vi "Data Manager.vi"(0 "Max Av Values In":dbl[](array[numeric]), 1 "Data Array In":dbl[][](array[numeric]), 3 "Data":dbl[](array[numeric]), 4 "Is PAT Test?":bool) -> (6 "Max Av Values Out":dbl[](array[numeric]), 7 "Data Array Out":dbl[][](array[numeric]))   [LabVIEW 2018]
uses:
  <vilib>/Analysis/baseanly.llb/Mean (DBL).vi
  <vilib>/Analysis/NI_AALBase.lvlib
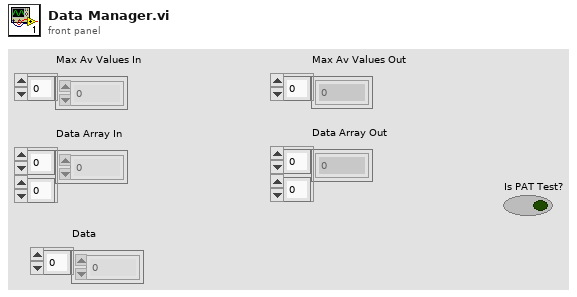
[diagram p1: front panel]
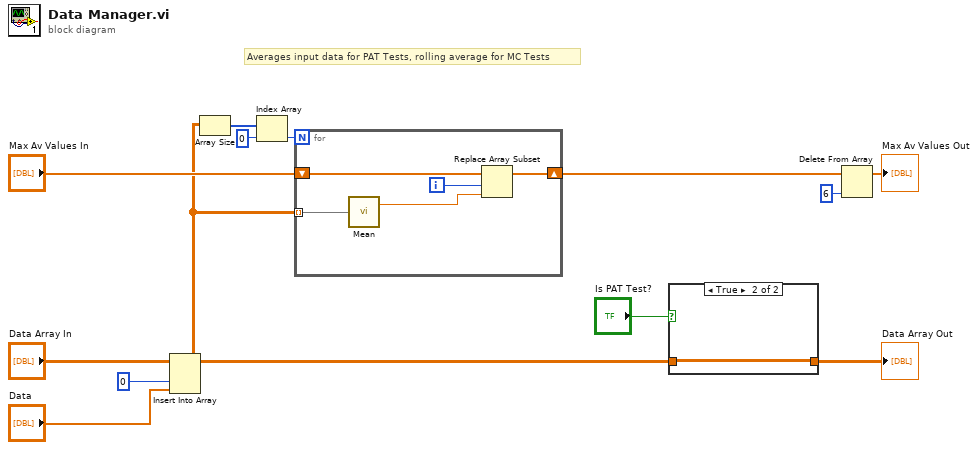
[diagram p0: block diagram]
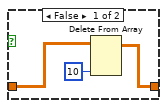
[diagram p2: hidden frame]
diagram:
  # "Averages input data for PAT Tests, rolling average for MC Tests"
  n1 = Insert Into Array(array="Data Array In", index (col)=0, new element="Data") -> (w3:dbl[][])  [unwired: 1 in]
  n2 = Array Size(array=w3) -> (size(s)=w12:i32[])
  n3 = Index Array(array=w12, index=0) -> (element=w13:i32)
  n4 = for {
    N: w13 -> [_]
    tunnel: w3 -> [w15] mode=indexing
    shift-right: [w17] -> w1
    shift-left: "Max Av Values In" -> [w18]
    i -> [w14]
    n5 = call-poly <vilib>:"Mean.vi"("X"=w15) -> ("mean"=w16:dbl)  [unwired: 1 out]
    n6 = Replace Array Subset(array=w18, new element=w16, index=w14) -> (w17:dbl[])
  }
  n7 = case shown="True" "Is PAT Test?" {
    tunnel: w3 -> [w21 w22]
    tunnel: [w19 w22] -> w2
    frame False {
      n8 = Delete From Array(array=w21, index (col)=10) -> (array with subset deleted=w19:dbl[][])  [unwired: 2 in, 1 out]
    }
    frame True {
    }
  }
  "Data Array Out" <- w2
  n9 = Delete From Array(array=w1, index=6) -> (array with subset deleted=→"Max Av Values Out":dbl[])  [unwired: 1 in, 1 out]
